vi "SendFFTStatusUpdateToBeckhoff.vi"(8 "error in (no error)":errorcluster, 10 "FFTStatusUpdateFlags":T1, 11 "Handle In":u32 format="%x") -> (0 "error out":errorcluster, 3 "Handle Out":u32 format="%x")   [LabVIEW 2020]
uses:
  <userlib>/Beckhoff-LabVIEW-Interface/_DependsOn/With TypeResolving/Write Sync Single TypeResolved.vi
panel:
  in  "WriteGrpSymbols 2":string[](array[string])=["192.168.0.20.1.1:851::GVL_LabviewDataShare.in_bAardvarkBoardError_labview", "192.168.0.20.1.1:851::GVL_LabviewDataShare.in_bAsic1CalibrationCompleted_labview", "192.168.0.20.1.1:851::GVL_LabviewDataShare.in_bAsic1CalibrationInProgress_labview", "192.168.0.20.1.1:851::GVL_LabviewDataShare.in_bAsic1CalibrationSuccess_labview", "192.168.0.20.1.1:851::GVL_LabviewDataShare.in_bAsic1FFTCompleted_labview", "192.168.0.20.1.1:851::GVL_LabviewDataShare.in_bAsic1FFTInProgress_labview", "192.168.0.20.1.1:851::GVL_LabviewDataShare.in_bAsic1FFTSuccess_labview", "192.168.0.20.1.1:851::GVL_LabviewDataShare.in_bAsic2CalibrationCompleted_labview", "192.168.0.20.1.1:851::GVL_LabviewDataShare.in_bAsic2CalibrationInProgress_labview", "192.168.0.20.1.1:851::GVL_LabviewDataShare.in_bAsic2CalibrationSuccess_labview", "192.168.0.20.1.1:851::GVL_LabviewDataShare.in_bAsic2FFTCompleted_labview", "192.168.0.20.1.1:851::GVL_LabviewDataShare.in_bAsic2FFTInProgress_labview", "192.168.0.20.1.1:851::GVL_LabviewDataShare.in_bAsic2FFTSuccess_labview", "192.168.0.20.1.1:851::GVL_LabviewDataShare.in_bCalResultsDBStoreSuccess_labview", "192.168.0.20.1.1:851::GVL_LabviewDataShare.in_bFFTResultsDBStoreSuccess_labview", "192.168.0.20.1.1:851::GVL_LabviewDataShare.in_bLabviewHandshakeBit", "192.168.0.20.1.1:851::GVL_LabviewDataShare.in_bLabviewResetComplete_labview", "192.168.0.20.1.1:851::GVL_LabviewDataShare.in_bLabviewResetSuccess_labview", "192.168.0.20.1.1:851::GVL_LabviewDataShare.in_bNIDaqError_labview", "192.168.0.20.1.1:851::GVL_LabviewDataShare.in_bPTC04BoardError_labview", "192.168.0.20.1.1:851::GVL_LabviewDataShare.in_bStartupInitializationCompleted_labview", "192.168.0.20.1.1:851::GVL_LabviewDataShare.in_bStartupInitializationSuccess_labview", "192.168.0.20.1.1:851::GVL_LabviewDataShare.in_strAsic1SerialNo_labview", "192.168.0.20.1.1:851::GVL_LabviewDataShare.in_strAsic2SerialNo_labview"]
  out "Write Status 4":bool
  out "Has Matched? 4":bool
  out "Write Status 3":bool
  out "Has Matched? 3":bool
  out "Write Status 2":bool
  out "Has Matched? 2":bool
  out "Write Status":bool
  out "Has Matched?":bool
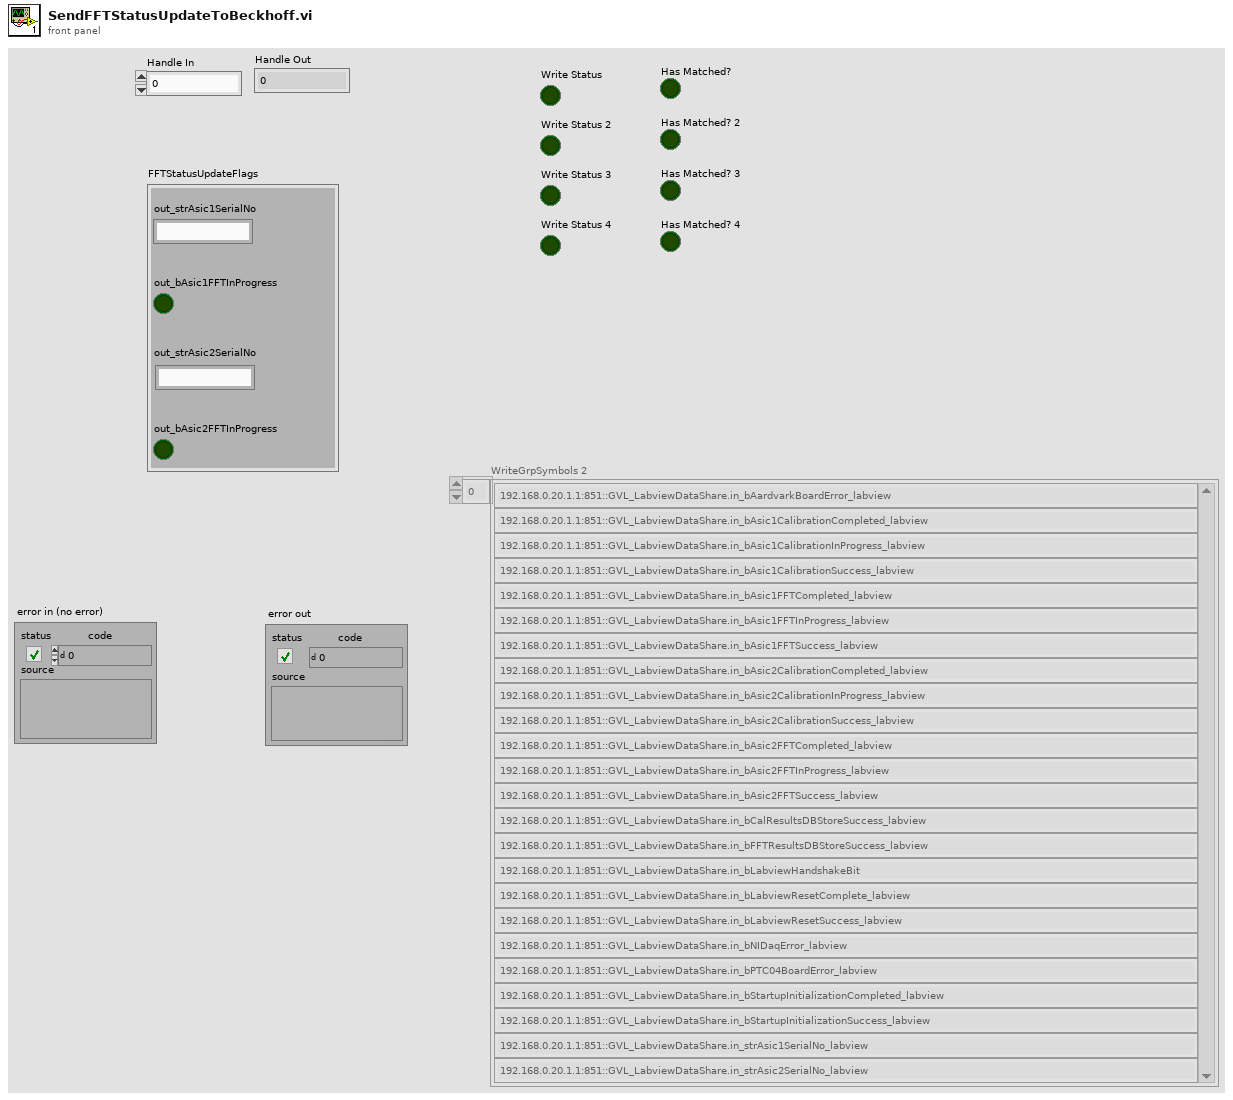
[diagram p1: front panel]
types:
  T1 = cluster{"out_strAsic1SerialNo":string, "out_bAsic1FFTInProgress":bool, "out_strAsic2SerialNo":string, "out_bAsic2FFTInProgress":bool}
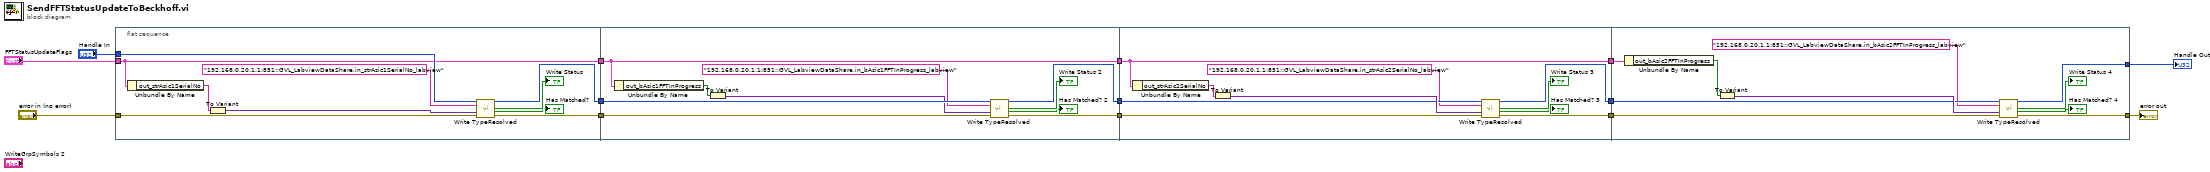
[diagram p0: block diagram]
diagram:
  n1 = flat-sequence {
    tunnel: "Handle In" -> [w24]
    tunnel: [w23] -> w14
    tunnel: [w22] -> w13
    tunnel: "error in (no error)" -> [w21]
    tunnel: "FFTStatusUpdateFlags" -> [w18]
    tunnel: [w18] -> w12
    tunnel: w14 -> [w34]
    tunnel: w13 -> [w33]
    tunnel: [w30] -> w11
    tunnel: [w29] -> w10
    tunnel: w12 -> [w28]
    tunnel: [w28] -> w9
    tunnel: [w41] -> w8
    tunnel: [w42] -> w7
    tunnel: w11 -> [w40]
    tunnel: w10 -> [w39]
    tunnel: w9 -> [w38]
    tunnel: [w38] -> w6
    tunnel: w8 -> [w51]
    tunnel: w7 -> [w52]
    tunnel: w6 -> [w50]
    tunnel: [w46] -> w3
    tunnel: [w45] -> w2
    frame #0 {
      n2 = Unbundle By Name(w18) -> ("out_strAsic1SerialNo"=w20:string)
      n3 = To Variant(anything=w20) -> (Variant=w19:variant)
      n4 = call-poly <userlib>:"Write TypeResolved.vi"("Handle"=w24, "SymbolName"="192.168.0.20.1.1:851::GVL_LabviewDataShare.in_strAsic1SerialNo_labview", "WData"=w19, "error constant"=w21) -> ("Handle"=w23:u32, "Write Status?"=→"Write Status":bool, "Has Matched?"=→"Has Matched?":bool, "error out"=w22:errorcluster)  [unwired: 8 in]
    }
    frame #1 {
      n5 = Unbundle By Name(w28) -> ("out_bAsic1FFTInProgress"=w32:bool)
      n6 = To Variant(anything=w32) -> (Variant=w31:variant)
      n7 = call-poly <userlib>:"Write TypeResolved.vi"("Handle"=w34, "SymbolName"="192.168.0.20.1.1:851::GVL_LabviewDataShare.in_bAsic1FFTInProgress_labview", "WData"=w31, "error constant"=w33) -> ("Handle"=w30:u32, "Write Status?"=→"Write Status 2":bool, "Has Matched?"=→"Has Matched? 2":bool, "error out"=w29:errorcluster)  [unwired: 8 in]
    }
    frame #2 {
      n8 = Unbundle By Name(w38) -> ("out_strAsic2SerialNo"=w44:string)
      n9 = To Variant(anything=w44) -> (Variant=w43:variant)
      n10 = call-poly <userlib>:"Write TypeResolved.vi"("Handle"=w40, "SymbolName"="192.168.0.20.1.1:851::GVL_LabviewDataShare.in_strAsic2SerialNo_labview", "WData"=w43, "error constant"=w39) -> ("Handle"=w41:u32, "Write Status?"=→"Write Status 3":bool, "Has Matched?"=→"Has Matched? 3":bool, "error out"=w42:errorcluster)  [unwired: 8 in]
    }
    frame #3 {
      n11 = Unbundle By Name(w50) -> ("out_bAsic2FFTInProgress"=w53:bool)
      n12 = To Variant(anything=w53) -> (Variant=w54:variant)
      n13 = call-poly <userlib>:"Write TypeResolved.vi"("Handle"=w51, "SymbolName"="192.168.0.20.1.1:851::GVL_LabviewDataShare.in_bAsic2FFTInProgress_labview", "WData"=w54, "error constant"=w52) -> ("Handle"=w46:u32, "Write Status?"=→"Write Status 4":bool, "Has Matched?"=→"Has Matched? 4":bool, "error out"=w45:errorcluster)  [unwired: 8 in]
    }
  }
  "error out" <- w2
  "Handle Out" <- w3
